vi "Add_Image_Position_Offset.vi"() -> (5 "Plug in titles":string[](array[string]), 7 "Plug in values":string[](array[string]))   [LabVIEW 2014]
uses:
  Globals/Meas_global.vi
  Globals/Trav_pos_global.vi
  Globals/Extra_Commands_Global.vi
  Utilities/Image acquisition and processing/Feature detection/Typedefs/ROI bounds.ctl
  Utilities/Image acquisition and processing/Feature detection/Typedefs/Theta range.ctl
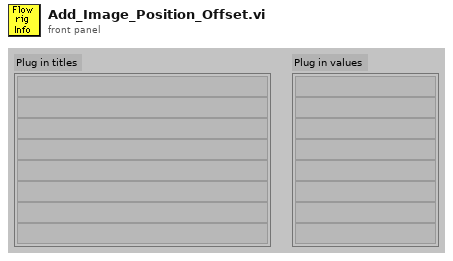
[diagram p1: front panel]
types:
  T1 = typedef "ROI bounds.ctl" = cluster{"Xmax":i32, "Ymax":i32, "Xmin":i32, "Ymin":i32}
  T2 = typedef "Theta range.ctl" = cluster{"theta max (deg)":dbl, "theta min (deg)":dbl}
  T3 = typedef "Traverse_cluster.ctl" = cluster{"Start X":sgl, "Start Y":sgl, "Start Z":sgl, "End X":sgl, "End Y":sgl, "End Z":sgl, "No. of pts.":i32, "Spacing":T4, "Filename":path, "Tunnel Speed":dbl, "Averaging time (min)":dbl, "Extra Commands":string, "Carrier_1 Q (l/min)":dbl, "Carrier_2 Q (l/min)":dbl, "Trace Gas Concentration (%)":dbl, "Specific Arguments":string, "Comments":string, "Row No":i32, "Row Type Selector":T5, "Completion time":string, "Row Duration (mins)":dbl, "No. of Valid pts.":i32, "Meas Setup File":string}
  T4 = typedef "Spacing.ctl" = enum16{"Linear", "Log", "Gauss", "Specified", "N/A"}
  T5 = typedef "Multi_run_mode.ctl" = enum16{"Move Traverse Only", "Set Tunnel Speed Only", "Set Source Only", "Set Measurement Conditions", "Single Measurement", "Vertical Profile", "Lateral Profile", "Longitudinal Profile", "Explore Volume", "Multi-Axis Profile", "Auto Calibrate", "Meas Fast FID Bkgnd", "Check Beam Power", "Scanning Valve Measurement", "Run VI Named:", "Set ADAM Ch", "Wait (minutes)", "Send Message", "Synchronize With:", "Fall Back to this Row", "Turn Off Row Repeating", "Blank Row", "Traverse 3D Volume"}
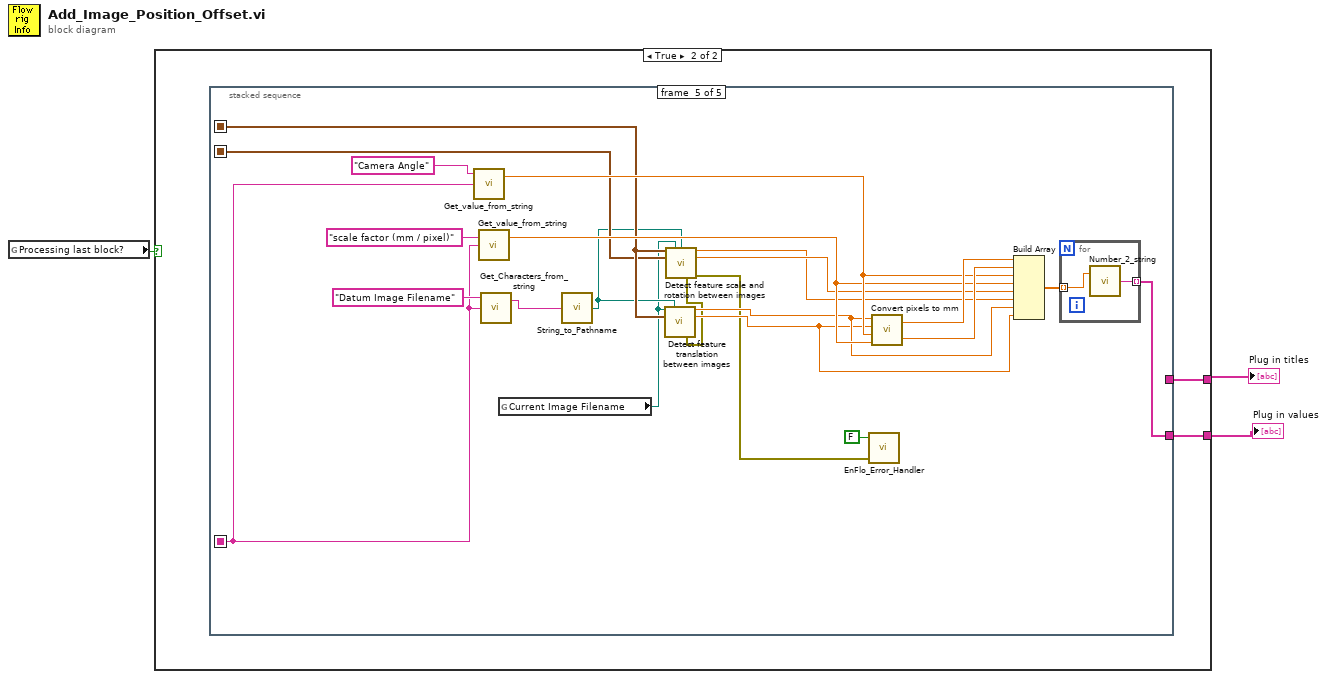
[diagram p0: block diagram]
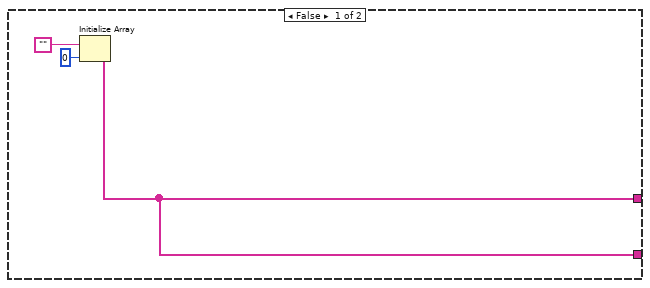
[diagram p2: hidden frame]
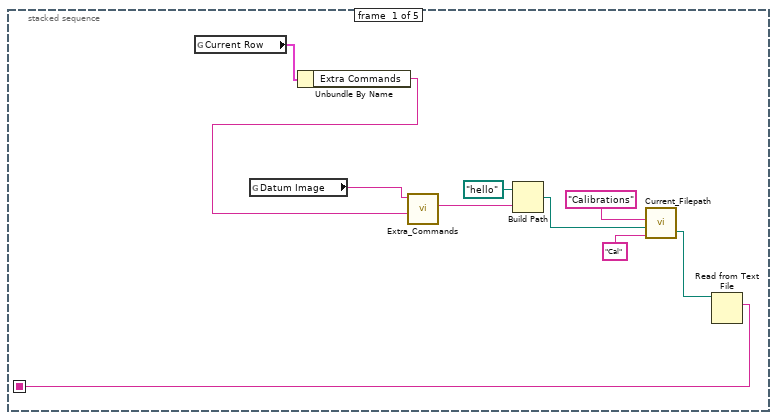
[diagram p3: hidden frame]
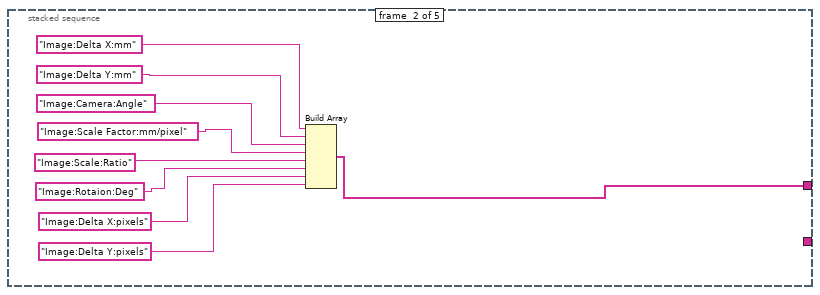
[diagram p4: hidden frame]
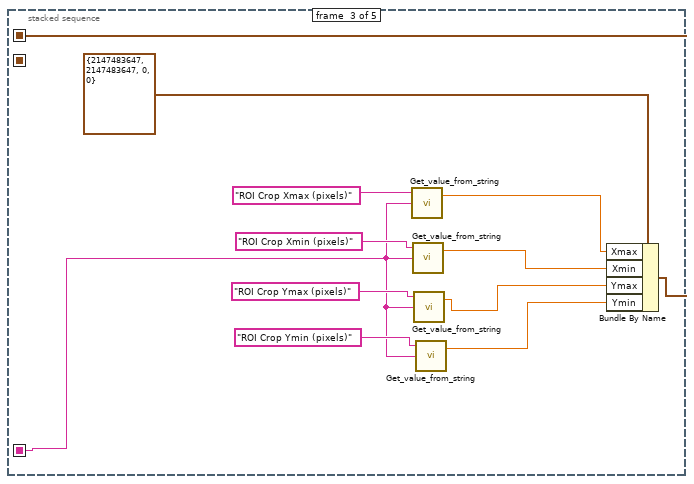
[diagram p5: hidden frame]
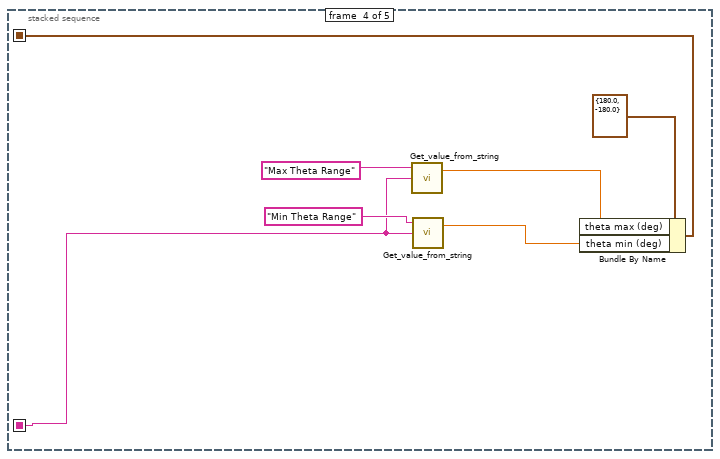
[diagram p6: hidden frame]
diagram:
  n1 = global read "Meas_global.vi" "Processing last block?"() -> (w3:bool)
  n2 = case shown="True" w3 {
    tunnel: [w4 w7] -> w2
    tunnel: [w4 w8] -> w1
    frame False {
      n3 = Initialize Array("", 0) -> (w4:string[])
    }
    frame True {
      n4 = stacked-sequence {
        seq-local: [w9 _ _ _ _] -> [_ _ w34 w43 w64]
        seq-local: [_ _ w28 _ _] -> [_ _ _ _ w56]
        seq-local: [_ _ _ w39 _] -> [_ _ _ _ w55]
        tunnel: [_ _ _ _ w57] -> w8
        tunnel: [_ w19 _ _ _] -> w7
        frame #0 {
          n5 = global read "Trav_pos_global.vi" "Current Row"() -> (w17:T3)
          n6 = global read "Extra_Commands_Global.vi" "Datum Image"() -> (w18:string)
          n7 = Unbundle By Name(w17) -> ("Extra Commands"=w16:string)
          n8 = call "Extra_Commands.vi"("String to Search"=w16, "Command"=w18) -> ("String Value"=w11:string)  [unwired: 1 in, 4 out]
          n9 = Build Path(base path=path "hello", name or relative path=w11) -> (appended path=w15:path)
          n10 = call "Current_Filepath.vi"("Short_Name"="Cal" ("Data Type"), "Filename in"=w15, "Data Type"="Calibrations") -> ("Filename Out"=w10:path)  [unwired: 1 in, 1 out]
          n11 = Read from Text File(file (use dialog)=w10) -> (text=w9:string)  [unwired: 3 in, 3 out]
        }
        frame #1 {
          n12 = Build Array("Image:Delta X:mm", "Image:Delta Y:mm", "Image:Camera:Angle", "Image:Scale Factor:mm/pixel", "Image:Scale:Ratio", "Image:Rotaion:Deg", "Image:Delta X:pixels", "Image:Delta Y:pixels") -> (w19:string[])
        }
        frame #2 {
          n13 = call "Get_value_from_string.vi"("Input string"=w34, "Variable name"="ROI Crop Xmax (pixels)" ("Label for characters")) -> ("Value"=w32:dbl)  [unwired: 1 in, 1 out]
          n14 = call "Get_value_from_string.vi"("Input string"=w34, "Variable name"="ROI Crop Xmin (pixels)" ("Label for characters")) -> ("Value"=w31:dbl)  [unwired: 1 in, 1 out]
          n15 = call "Get_value_from_string.vi"("Input string"=w34, "Variable name"="ROI Crop Ymax (pixels)" ("Label for characters")) -> ("Value"=w30:dbl)  [unwired: 1 in, 1 out]
          n16 = call "Get_value_from_string.vi"("Input string"=w34, "Variable name"="ROI Crop Ymin (pixels)" ("Label for characters")) -> ("Value"=w29:dbl)  [unwired: 1 in, 1 out]
          n17 = Bundle By Name(cluster=T1 {"Xmax"=2147483647, "Ymax"=2147483647, "Xmin"=0, "Ymin"=0} ("ROI to crop (pixels)"), "Xmax"=w32, "Xmin"=w31, "Ymax"=w30, "Ymin"=w29) -> (w28:T1)
        }
        frame #3 {
          n18 = call "Get_value_from_string.vi"("Input string"=w43, "Variable name"="Max Theta Range" ("Label for characters")) -> ("Value"=w42:dbl)  [unwired: 1 in, 1 out]
          n19 = call "Get_value_from_string.vi"("Input string"=w43, "Variable name"="Min Theta Range" ("Label for characters")) -> ("Value"=w41:dbl)  [unwired: 1 in, 1 out]
          n20 = Bundle By Name(cluster=T2 {"theta max (deg)"=180.0, "theta min (deg)"=-180.0} ("Theta range (deg)"), "theta max (deg)"=w42, "theta min (deg)"=w41) -> (w39:T2)
        }
        frame #4 {
          n21 = call "Get_value_from_string.vi"("Input string"=w64, "Variable name"="Camera Angle" ("Label for value")) -> ("Value"=w60:dbl)  [unwired: 1 in, 1 out]
          n22 = call "Get_value_from_string.vi"("Input string"=w64, "Variable name"="scale factor (mm / pixel)" ("Label for value")) -> ("Value"=w59:dbl)  [unwired: 1 in, 1 out]
          n23 = call "Get_Characters_from_string.vi"("Input string"=w64, "Variable name"="Datum Image Filename" ("Label for characters")) -> ("Value"=w63:string)  [unwired: 1 in, 1 out]
          n24 = global read "Trav_pos_global.vi" "Current Image Filename"() -> (w49:path)
          n25 = call "String_to_Pathname.vi"("Input String"=w63) -> ("path"=w50:path)
          n26 = call "Detect feature translation between images.vi"("Test image file path"=w49, "Reference image file path"=w50, "ROI to crop (pixels)"=w56) -> ("dx (pix)"=w52:dbl, "dy (pix)"=w51:dbl, "Error out"=w48:errorcluster)  [unwired: 8 in, 2 out]
          n27 = call "Detect feature scale and rotation between images.vi"("ROI to crop (pixels)"=w56, "Test image file path"=w49, "Reference image file path"=w50, "Theta range (deg)"=w55, "Error In"=w48) -> ("Rotation (deg)"=w53:dbl, "Scale factor"=w54:dbl, "Error out"=w47:errorcluster)  [unwired: 6 in, 2 out]
          n28 = call "EnFlo_Error_Handler.vi"("error in (no error)"=w47, "Dialog Box (T)"=FALSE) -> ()  [unwired: 1 in, 3 out]
          n29 = call "Convert pixels to mm.vi"("scale factor (mm / pixel)"=w59, "camera angle, ccw+ rel. to trav. (deg)"=w60, "dy (pix)"=w51, "dx (pix)"=w52) -> ("dy (mm)"=w61:dbl, "dx (mm)"=w62:dbl)
          n30 = Build Array(w62, w61, w60, w59, w54, w53, w52, w51) -> (w58:dbl[])
          n31 = for {
            tunnel: w58 -> [w69] mode=indexing
            tunnel: [w68] -> w57 mode=indexing
            n32 = call "Number_2_string.vi"("number"=w69) -> ("String"=w68:string)  [unwired: 1 in]
          }
        }
      }
    }
  }
  "Plug in titles" <- w2
  "Plug in values" <- w1
